vi "Read Name.vi"(0 "controller in":refnum<class "Generic Plugin.lvclass">, 1 "error in (no error)":errorcluster) -> (2 "controller out":refnum<class "Generic Plugin.lvclass">, 3 "Name":string, 4 "error out":errorcluster)   [LabVIEW 2020, in "Generic Plugin.lvclass"]
uses:
  Generic Plugin.lvclass
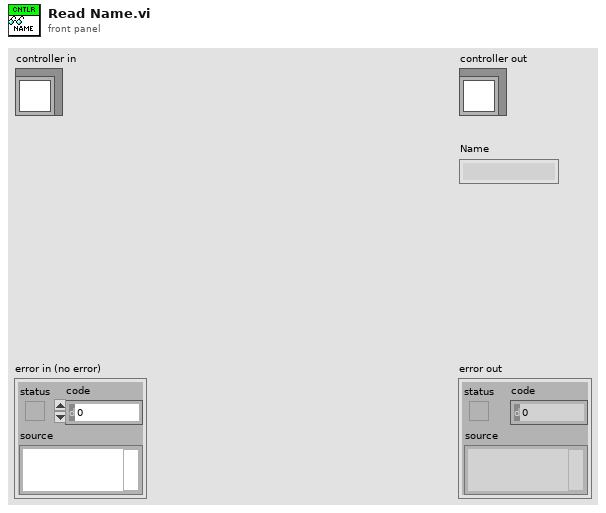
[diagram p1: front panel]
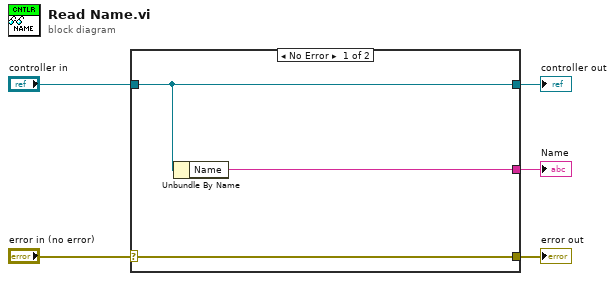
[diagram p0: block diagram]
diagram:
  n1 = case shown="No Error" "error in (no error)" {
    selector: "error in (no error)" -> [w8 w9]
    tunnel: [w8 w9] -> w4
    tunnel: [w7 w10] -> w2
    tunnel: "controller in" -> [w7 w10]
    tunnel: [w6 _] -> w1
    frame No Error {
      n2 = Unbundle By Name(w7) -> ("Name"=w6:string)
    }
    frame Error {
    }
  }
  "error out" <- w4
  "controller out" <- w2
  "Name" <- w1
